vi "minicryo_Harry-IcH - v6.vi"(6 "Mag Field Step":dbl=0.002, 7 "Directory Output":string="C:\\User Data\\hlb54\\210111_42B\\JJ1\\IcH_pos_to_neg_T=4p00K_set=0p0T", 8 "Stop Field":dbl=-0.2, 9 "Start Field (T)":dbl=0.2 format="%#_7f", 10 "Stop":bool, 11 "Measure":bool) -> ()   [LabVIEW 2013]
uses:
  Global 2.vi
  B_Globals.vi
  <vilib>/Utility/file.llb/Read From Spreadsheet File (DBL).vi
panel:
  out "Sample Temp [K] - Meas":dbl=8.00109
  out "dV/dI-I":cluster{dbl[], dbl[]}(graph) caption="XY Graph"
  out "I-V":cluster{dbl[], dbl[]}(graph) caption="XY Graph"
  out "Status":string="Welcome!"
  in  "Keithley":refnum<visa-resource-name>="GPIB0::20::INSTR"
  in  "Delay [sec]":dbl=0.002 format="%#_6e"
  in  "Compliance [V] 2":dbl=10.0 format="%#_6f"
  in  "Delta [A]":dbl=1e-05 format="%#_6e"
  in  "Abort Conductance":bool
  in  "Step [A]":dbl=2e-05 format="%#_6e"
  in  "I-Max [A]":dbl=0.015 format="%#_6e"
  in  "Arm Conductance":bool
  out "B Now":string="-0.202"
  out "error out 6":errorcluster
  in  "Minicryo":bool=TRUE
  in  "Field and rate":dbl[][](array[numeric])
  in  "step":bool=TRUE
  in  "Set Rate (T/min)":dbl=0.1
  out "?":refnum<visa-resource-name>="GPIB0::20::INSTR"
  out "Iteration?":i32=401
  out "B Aim":dbl=-0.202
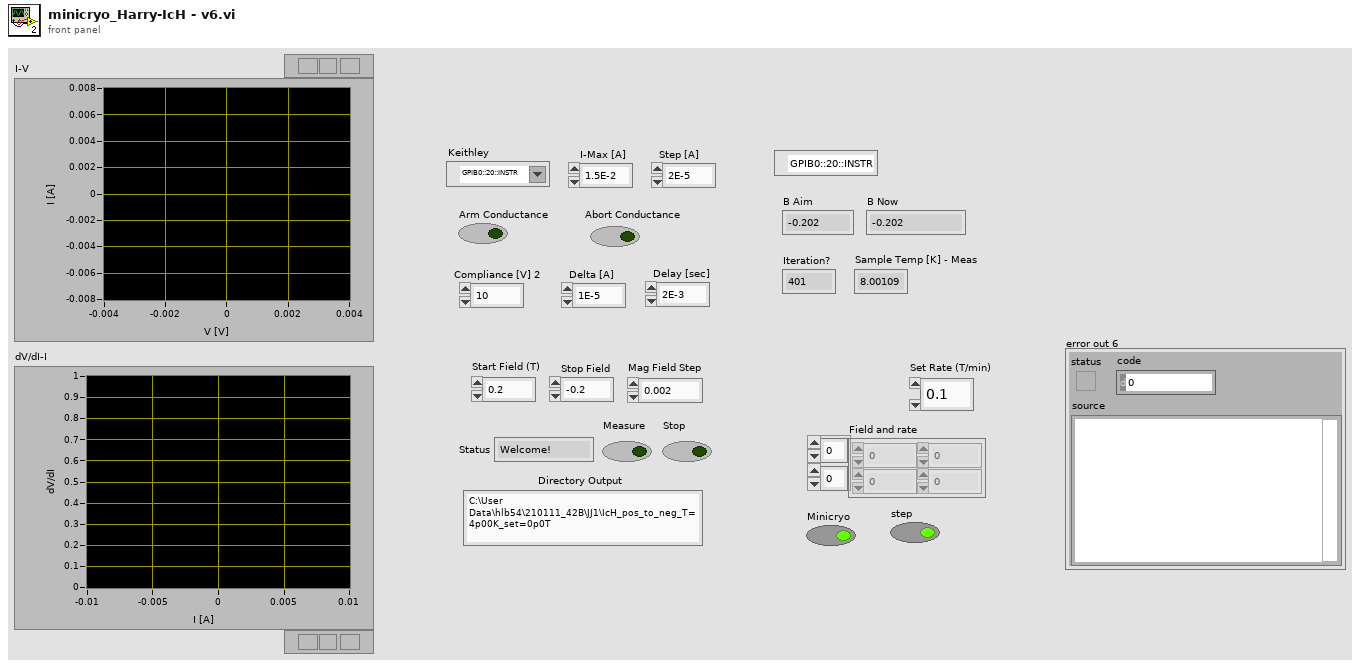
[diagram p1: front panel]
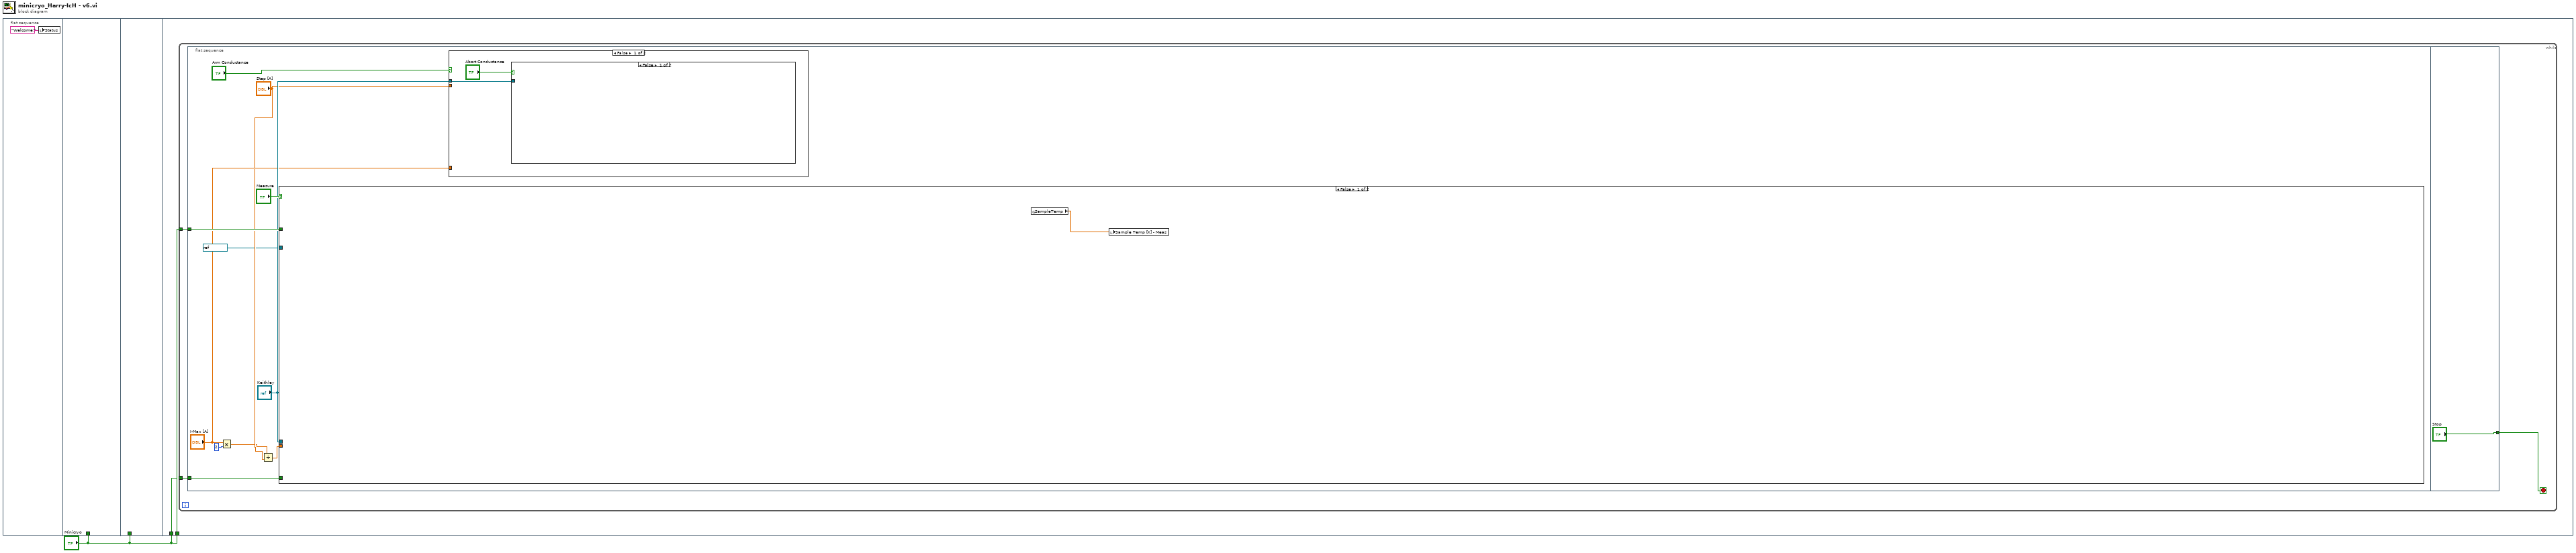
[diagram p0: block diagram]
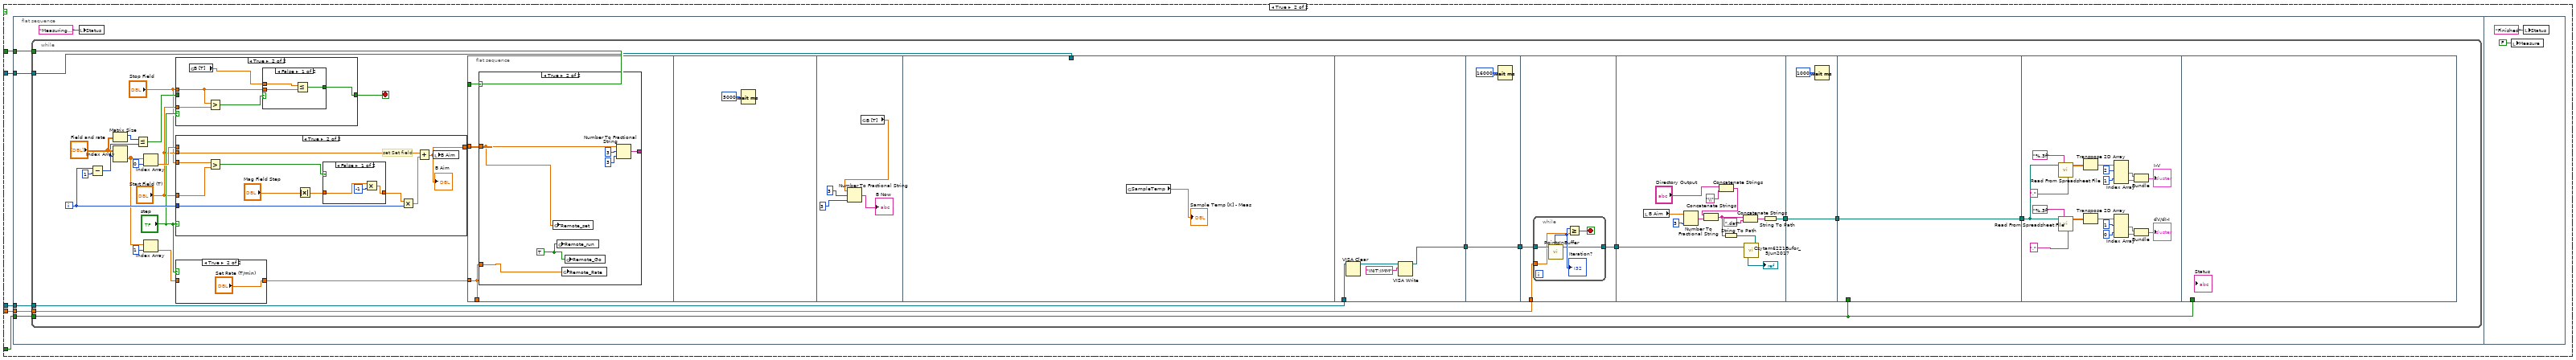
[diagram p2: hidden frame]
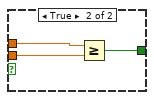
[diagram p4: hidden frame]
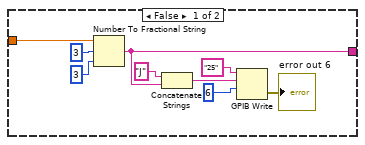
[diagram p8: hidden frame]
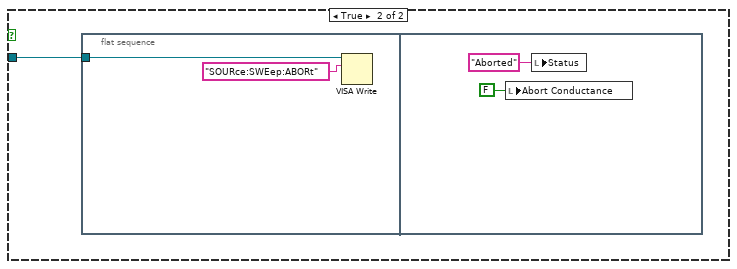
[diagram p9: hidden frame]
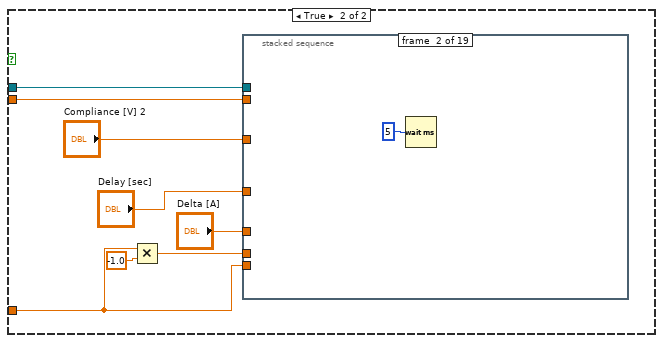
[diagram p10: hidden frame]
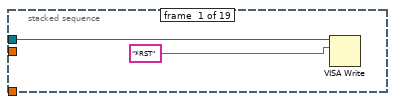
[diagram p11: hidden frame]
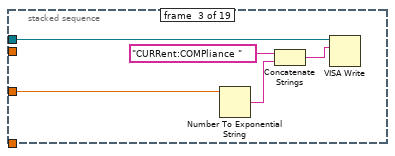
[diagram p12: hidden frame]
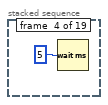
[diagram p13: hidden frame]
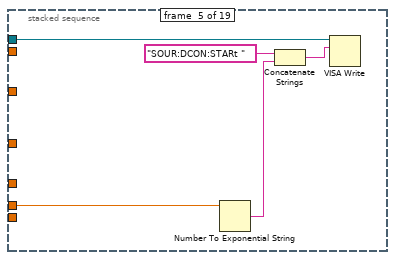
[diagram p14: hidden frame]
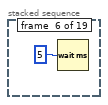
[diagram p15: hidden frame]
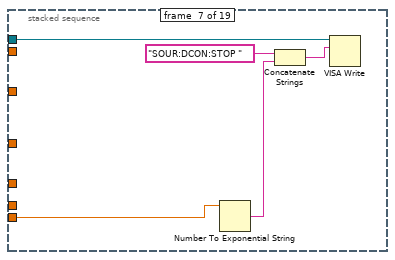
[diagram p16: hidden frame]
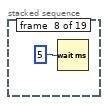
[diagram p17: hidden frame]
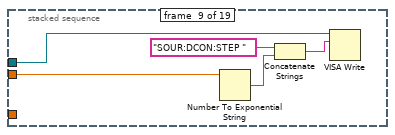
[diagram p18: hidden frame]
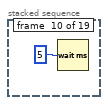
[diagram p19: hidden frame]
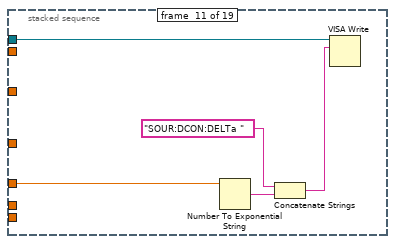
[diagram p20: hidden frame]
diagram:
  n1 = flat-sequence {
    tunnel: "Minicryo" -> [_]
    tunnel: "Minicryo" -> [_]
    tunnel: "Minicryo" -> [w4]
    tunnel: "Minicryo" -> [w3]
    frame #0 {
      n2 = local write "Status"("Welcome!") -> ()
    }
    frame #1 {
    }
    frame #2 {
    }
    frame #3 {
      n3 = while {
        tunnel: w4 -> [w7]
        tunnel: w3 -> [w6]
        stop <- w5 stop-if-true
        n4 = flat-sequence {
          tunnel: w7 -> [w18]
          tunnel: w6 -> [w17]
          tunnel: ["Stop"] -> w5
          frame #0 {
            n5 = Multiply(x="I-Max [A]", y=2) -> (x*y=w9:dbl)
            n6 = Divide(x=w9, y="Step [A]") -> (x/y=w10:dbl)
            n7 = case shown="False" "Measure" {
              tunnel: w18 -> [_ w24]
              tunnel: w17 -> [_ w23]
              tunnel: "Keithley" -> [_ w22]
              tunnel: w10 -> [_ w21]
              tunnel: refnum<visa-resource-name> "COM7" ("LakeShore340") -> [_ w20]
              frame False {
                n8 = global read "Global 2.vi" "SampleTemp"() -> (w19:dbl)
                n9 = local write "Sample Temp [K] - Meas"(w19) -> ()
              }
              frame True {
                n10 = flat-sequence {
                  tunnel: w24 -> [w30]
                  tunnel: w23 -> [w29]
                  tunnel: w22 -> [w28]
                  tunnel: w21 -> [w27]
                  tunnel: w20 -> [w25]
                  frame #0 {
                    n11 = while {
                      tunnel: w30 -> [w46]
                      tunnel: w29 -> [w41]
                      tunnel: w28 -> [w39]
                      tunnel: w27 -> [w38]
                      tunnel: w25 -> [w31]
                      i -> [w52]
                      stop <- w37 stop-if-true
                      n12 = Subtract(x=w52, y=1) -> (x-y=w43:i32)
                      n13 = Matrix Size(0:"Field and rate") -> (1:w44:i32)  [unwired: 1 out]
                      n14 = Index Array(array="Field and rate", index (row)=w43) -> (element=w49:dbl[])  [unwired: 1 in]
                      n15 = Less Or Equal?(x=w44, y=w43) -> (x <= y?=w42:bool)
                      n16 = Index Array(array=w49, index=0) -> (element=w48:dbl)
                      n17 = Index Array(array=w49, index=1) -> (element=w47:dbl)
                      n18 = case shown="True" "step" {
                        tunnel: [w59 w64] -> w37
                        tunnel: w42 -> [w59 _]
                        tunnel: "Stop Field" -> [_ w63]
                        tunnel: "Start Field (T)" -> [_ w62]
                        frame False {
                        }
                        frame True {
                          n19 = global read "B_Globals.vi" "B [T]"() -> (w60:dbl)
                          n20 = Greater?(x=w63, y=w62) -> (0:w61:bool)
                          n21 = case shown="False" w61 {
                            tunnel: [w67 w70] -> w64
                            tunnel: w60 -> [w65 w69]
                            tunnel: w63 -> [w66 w68]
                            frame False {
                              n22 = Less Or Equal?(x=w65, y=w66) -> (x <= y?=w67:bool)
                            }
                            frame True {
                              n23 = Greater Or Equal?(x=w69, y=w68) -> (x >= y?=w70:bool)
                            }
                          }
                        }
                      }
                      n24 = case shown="True" "step" {
                        tunnel: [w73 w82] -> w58
                        tunnel: w52 -> [_ w81]
                        tunnel: w48 -> [w73 _]
                        tunnel: "Start Field (T)" -> [_ w80]
                        tunnel: "Start Field (T)" -> [_ w79]
                        tunnel: "Stop Field" -> [_ w78]
                        frame False {
                        }
                        frame True {
                          # "set Set field"
                          n25 = Greater?(x=w78, y=w79) -> (0:w74:bool)
                          n26 = Absolute Value(x="Mag Field Step") -> (abs(x)=w76:dbl)
                          n27 = case shown="False" w74 {
                            tunnel: [w86 w87] -> w75
                            tunnel: w76 -> [w84 w87]
                            frame False {
                              n28 = Multiply(x=w84, y=-1) -> (x*y=w86:dbl)
                            }
                            frame True {
                            }
                          }
                          n29 = Multiply(x=w75, y=w81) -> (x*y=w83:dbl)
                          n30 = Add(x=w80, y=w83) -> (x+y=w82:dbl)
                          "B Aim" <- w82
                          n31 = local write "B Aim"(w82) -> ()
                        }
                      }
                      n32 = case shown="True" "step" {
                        tunnel: [w71 "Set Rate (T/min)"] -> w54
                        tunnel: w47 -> [w71 _]
                        frame False {
                        }
                        frame True {
                        }
                      }
                      n33 = flat-sequence {
                        tunnel: w58 -> [w90]
                        tunnel: [w89] -> _
                        tunnel: w54 -> [w89]
                        tunnel: w46 -> [w88]
                        tunnel: w31 -> [_]
                        tunnel: [w113] -> w56
                        tunnel: w39 -> [w112]
                        tunnel: [w117] -> w57
                        tunnel: w56 -> [w117]
                        tunnel: w57 -> [w120]
                        tunnel: [w119] -> w55
                        tunnel: w38 -> [w118]
                        tunnel: w55 -> [w133]
                        tunnel: [w129] -> w32
                        tunnel: [w139] -> w33
                        tunnel: w32 -> [w139]
                        tunnel: w41 -> [_]
                        tunnel: [w141] -> w34
                        tunnel: w33 -> [w141]
                        tunnel: w34 -> [w142]
                        tunnel: w41 -> [_]
                        frame #0 {
                          n34 = case shown="True" w88 {
                            tunnel: w90 -> [w93 w100]
                            tunnel: w89 -> [_ w102]
                            tunnel: [w91 w103] -> _
                            frame False {
                              n35 = Number To Fractional String(number=w93, width (-)=i16 3, precision (6)=i16 3) -> (F-format string=w91:string)  [unwired: 1 in]
                              n36 = Concatenate Strings("J" ("string"), w91) -> (w92:string)
                              n37 = GPIB Write(0:"25" ("address string"), 1:w92, 2:6) -> (6:→"error out 6":errorcluster)  [unwired: 2 in, 1 out]
                            }
                            frame True {
                              w101 = TRUE
                              n38 = global write "B_Globals.vi" "Remote_set"(w100) -> ()
                              n39 = global write "B_Globals.vi" "Remote_run"(w101) -> ()
                              n40 = global write "B_Globals.vi" "Remote_Rate"(w102) -> ()
                              n41 = global write "B_Globals.vi" "Remote_Go"(w101) -> ()
                              n42 = Number To Fractional String(number=w100, width (-)=i16 3, precision (6)=i16 3) -> (F-format string=w103:string)  [unwired: 1 in]
                            }
                          }
                        }
                        frame #1 {
                          n43 = Wait (ms)(milliseconds to wait=u32 5000) -> ()  [unwired: 1 out]
                        }
                        frame #2 {
                          n44 = global read "B_Globals.vi" "B [T]"() -> (w107:dbl)
                          n45 = Number To Fractional String(number=w107, width (-)=i16 3, precision (6)=i16 3) -> (F-format string=→"B Now":string)  [unwired: 1 in]
                        }
                        frame #3 {
                          n46 = global read "Global 2.vi" "SampleTemp"() -> (→"Sample Temp [K] - Meas":dbl)
                        }
                        frame #4 {
                          n47 = VISA Clear(VISA resource name=w112) -> (VISA resource name out=w115:refnum<visa-resource-name>)  [unwired: 1 in, 1 out]
                          n48 = VISA Write(VISA resource name=w115, write buffer="INIT:IMM") -> (VISA resource name out=w113:refnum<visa-resource-name>)  [unwired: 1 in, 2 out]
                        }
                        frame #5 {
                          n49 = Wait (ms)(milliseconds to wait=16000) -> ()  [unwired: 1 out]
                        }
                        frame #6 {
                          n50 = while {
                            tunnel: w120 -> [w123]
                            tunnel: [w122] -> w119
                            tunnel: w118 -> [w121]
                            stop <- w124 stop-if-true
                            n51 = call "PointsInBuffer.vi"("VISA resource name"=w123) -> (3:w122:refnum<visa-resource-name>, "number"=w125:i32)  [unwired: 9 in]
                            "Iteration?" <- w125
                            n52 = Greater Or Equal?(x=w125, y=w121) -> (x >= y?=w124:bool)
                          }
                        }
                        frame #7 {
                          n53 = local read "B Aim"() -> (w134:dbl)
                          n54 = Number To Fractional String(number=w134, precision (6)=i16 3) -> (F-format string=w138:string)  [unwired: 2 in]
                          n55 = Concatenate Strings("Directory Output", "\\") -> (w126:string)
                          n56 = Concatenate Strings(w126, w138) -> (w131:string)
                          n57 = String To Path(string=w131) -> (path=w137:path)
                          n58 = Concatenate Strings(w131, ".dat") -> (w130:string)
                          n59 = call "Czytam6221Bufor_5Jun2017.vi"("file path (dialog if empty)"=w137, 3:w133) -> (2:→"?":refnum<visa-resource-name>)  [unwired: 1 in]
                          n60 = String To Path(string=w130) -> (path=w129:path)
                        }
                        frame #8 {
                          n61 = Wait (ms)(milliseconds to wait=u32 1000) -> ()  [unwired: 1 out]
                        }
                        frame #9 {
                        }
                        frame #10 {
                          n62 = call-poly <vilib>:"Read From Spreadsheet File.vi"("delimiter (\\t)"="," ("delimiter (\\t)"), "format (%.3f)"="%.3f", "file path (dialog if empty)"=w142) -> ("all rows"=w155:dbl[][])  [unwired: 4 in, 4 out]
                          n63 = call-poly <vilib>:"Read From Spreadsheet File.vi"("delimiter (\\t)"="," ("delimiter (\\t)"), "format (%.3f)"="%.3f", "file path (dialog if empty)"=w142) -> ("all rows"=w146:dbl[][])  [unwired: 4 in, 4 out]
                          n64 = Transpose 2D Array(2D array=w155) -> (transposed array=w154:dbl[][])
                          n65 = Transpose 2D Array(2D array=w146) -> (transposed array=w145:dbl[][])
                          n66 = Index Array(array=w154, index (row) #1=2 ("index (row)"), index (row) #2=1 ("index (row)")) -> (element #1=w157:dbl[], element #2=w156:dbl[])  [unwired: 2 in]
                          n67 = Index Array(array=w145, index (row) #1=1 ("index (row)"), index (row) #2=0 ("index (row)")) -> (element #1=w148:dbl[], element #2=w147:dbl[])  [unwired: 2 in]
                          n68 = Bundle(w157, w156) -> (→"I-V":cluster{dbl[], dbl[]})  [unwired: 1 in]
                          n69 = Bundle(w148, w147) -> (→"dV/dI-I":cluster{dbl[], dbl[]})  [unwired: 1 in]
                        }
                        frame #11 {
                        }
                      }
                    }
                    n70 = local write "Status"("Measuring...") -> ()
                  }
                  frame #1 {
                    n71 = local write "Measure"(FALSE) -> ()
                    n72 = local write "Status"("Finished") -> ()
                  }
                }
              }
            }
            n73 = case shown="False" "Arm Conductance" {
              tunnel: "Keithley" -> [w163 w173]
              tunnel: "Step [A]" -> [_ w172]
              tunnel: "I-Max [A]" -> [_ w170]
              frame False {
                n74 = case shown="False" "Abort Conductance" {
                  tunnel: w163 -> [_ w165]
                  frame False {
                  }
                  frame True {
                    n75 = flat-sequence {
                      tunnel: w165 -> [w166]
                      frame #0 {
                        n76 = VISA Write(VISA resource name=w166, write buffer="SOURce:SWEep:ABORt") -> ()  [unwired: 1 in, 3 out]
                      }
                      frame #1 {
                        n77 = local write "Abort Conductance"(FALSE) -> ()
                        n78 = local write "Status"("Aborted") -> ()
                      }
                    }
                  }
                }
              }
              frame True {
                n79 = Multiply(x=w170, y=-1.0) -> (x*y=w171:dbl)
                n80 = stacked-sequence {
                  tunnel: w171 -> [_ _ _ _ w189 _ _ _ _ _ _ _ _ _ _ _ _ _ _]
                  tunnel: "Delay [sec]" -> [_ _ _ _ _ _ _ _ _ _ _ _ w212 _ _ _ _ _ _]
                  tunnel: "Compliance [V] 2" -> [_ _ w182 _ _ _ _ _ _ _ _ _ _ _ _ _ _ _ _]
                  tunnel: "Delta [A]" -> [_ _ _ _ _ _ _ _ _ _ w206 _ _ _ _ _ _ _ _]
                  tunnel: w173 -> [w179 _ w181 _ w187 _ w194 _ w200 _ w205 _ w211 _ w217 _ w220 _ _]
                  tunnel: w172 -> [_ _ _ _ _ _ _ _ w199 _ _ _ _ _ _ _ _ _ _]
                  tunnel: w170 -> [_ _ _ _ _ _ w193 _ _ _ _ _ _ _ _ _ _ _ _]
                  frame #0 {
                    n81 = VISA Write(VISA resource name=w179, write buffer="*RST") -> ()  [unwired: 1 in, 3 out]
                  }
                  frame #1 {
                    n82 = Wait (ms)(milliseconds to wait=5) -> ()  [unwired: 1 out]
                  }
                  frame #2 {
                    n83 = Number To Exponential String(number=w182) -> (E-format string=w184:string)  [unwired: 3 in]
                    n84 = Concatenate Strings("CURRent:COMPliance ", w184) -> (w183:string)
                    n85 = VISA Write(VISA resource name=w181, write buffer=w183) -> ()  [unwired: 1 in, 3 out]
                  }
                  frame #3 {
                    n86 = Wait (ms)(milliseconds to wait=5) -> ()  [unwired: 1 out]
                  }
                  frame #4 {
                    n87 = Number To Exponential String(number=w189) -> (E-format string=w190:string)  [unwired: 3 in]
                    n88 = Concatenate Strings("SOUR:DCON:STARt ", w190) -> (w188:string)
                    n89 = VISA Write(VISA resource name=w187, write buffer=w188) -> ()  [unwired: 1 in, 3 out]
                  }
                  frame #5 {
                    n90 = Wait (ms)(milliseconds to wait=5) -> ()  [unwired: 1 out]
                  }
                  frame #6 {
                    n91 = Number To Exponential String(number=w193) -> (E-format string=w196:string)  [unwired: 3 in]
                    n92 = Concatenate Strings("SOUR:DCON:STOP ", w196) -> (w195:string)
                    n93 = VISA Write(VISA resource name=w194, write buffer=w195) -> ()  [unwired: 1 in, 3 out]
                  }
                  frame #7 {
                    n94 = Wait (ms)(milliseconds to wait=5) -> ()  [unwired: 1 out]
                  }
                  frame #8 {
                    n95 = Number To Exponential String(number=w199) -> (E-format string=w202:string)  [unwired: 3 in]
                    n96 = Concatenate Strings("SOUR:DCON:STEP ", w202) -> (w201:string)
                    n97 = VISA Write(VISA resource name=w200, write buffer=w201) -> ()  [unwired: 1 in, 3 out]
                  }
                  frame #9 {
                    n98 = Wait (ms)(milliseconds to wait=5) -> ()  [unwired: 1 out]
                  }
                  frame #10 {
                    n99 = Number To Exponential String(number=w206) -> (E-format string=w208:string)  [unwired: 3 in]
                    n100 = Concatenate Strings("SOUR:DCON:DELTa ", w208) -> (w207:string)
                    n101 = VISA Write(VISA resource name=w205, write buffer=w207) -> ()  [unwired: 1 in, 3 out]
                  }
                  frame #11 {
                    n102 = Wait (ms)(milliseconds to wait=5) -> ()  [unwired: 1 out]
                  }
                  frame #12 {
                    n103 = Number To Exponential String(number=w212) -> (E-format string=w214:string)  [unwired: 3 in]
                    n104 = Concatenate Strings("SOUR:DCON:DELay ", w214) -> (w213:string)
                    n105 = VISA Write(VISA resource name=w211, write buffer=w213) -> ()  [unwired: 1 in, 3 out]
                  }
                  frame #13 {
                    n106 = Wait (ms)(milliseconds to wait=5) -> ()  [unwired: 1 out]
                  }
                  frame #14 {
                    n107 = VISA Write(VISA resource name=w217, write buffer="UNIT OHMS ") -> ()  [unwired: 1 in, 3 out]
                  }
                  frame #15 {
                    n108 = Wait (ms)(milliseconds to wait=5) -> ()  [unwired: 1 out]
                  }
                  frame #16 {
                    n109 = VISA Write(VISA resource name=w220, write buffer="SOUR:DCON:ARM ") -> ()  [unwired: 1 in, 3 out]
                  }
                  frame #17 {
                    n110 = Wait (ms)(milliseconds to wait=3000) -> ()  [unwired: 1 out]
                  }
                  frame #18 {
                    n111 = local write "Arm Conductance"(FALSE) -> ()
                    n112 = local write "Status"("Armed") -> ()
                  }
                }
              }
            }
          }
          frame #1 {
          }
        }
      }
    }
  }
